vi "eodrecorder_modified.vi"() -> ()   [LabVIEW 2012]
uses:
  eodrecorderstates.ctl
  <vilib>/Utility/error.llb/DialogType.ctl
  <vilib>/_DAQmxBase/Internals/DAQmxBase Create Channel (AI-Voltage-Basic).vi
  <vilib>/_DAQmxBase/Internals/DAQmxBase Timing (Sample Clock).vi
  <vilib>/_DAQmxBase/Internals/DAQmxBase Read (Analog 2D DBL NChan NSamp).vi
panel:
  in  "Channel":tag="Dev1/ai0"
  out "String 2":string
  out "String":string
  out "Tab Control":enum32{"Live Data", "Edit Data", "View Data"}(tab)
  out "WaveformData":T1
  out "# Pretrigger Samples\nAcquired":i32
  out "Pre-Trigger Error Indicator":bool caption="Error Indicator\n(Indicates if trigger occurs before\npre-trigger samples were acquired)"
  in  "Channel Index":i32
  in  "Samples to Read":i32=1000 caption="Samples to Read per Iterartion"
  in  "Pretrigger Samples":i32
  in  "Threshold":dbl
  out "Waveform Graph":dbl[][](graph) caption="Measurement"
  in  "SampleRate":dbl=10000.0
  in  "LiveDataMode":bool
  in  "NumSamptoGrab":i32
  in  "Capture":bool
  in  "Stop":bool
  in  "Open Data":bool
  # "Off"
  # "On"
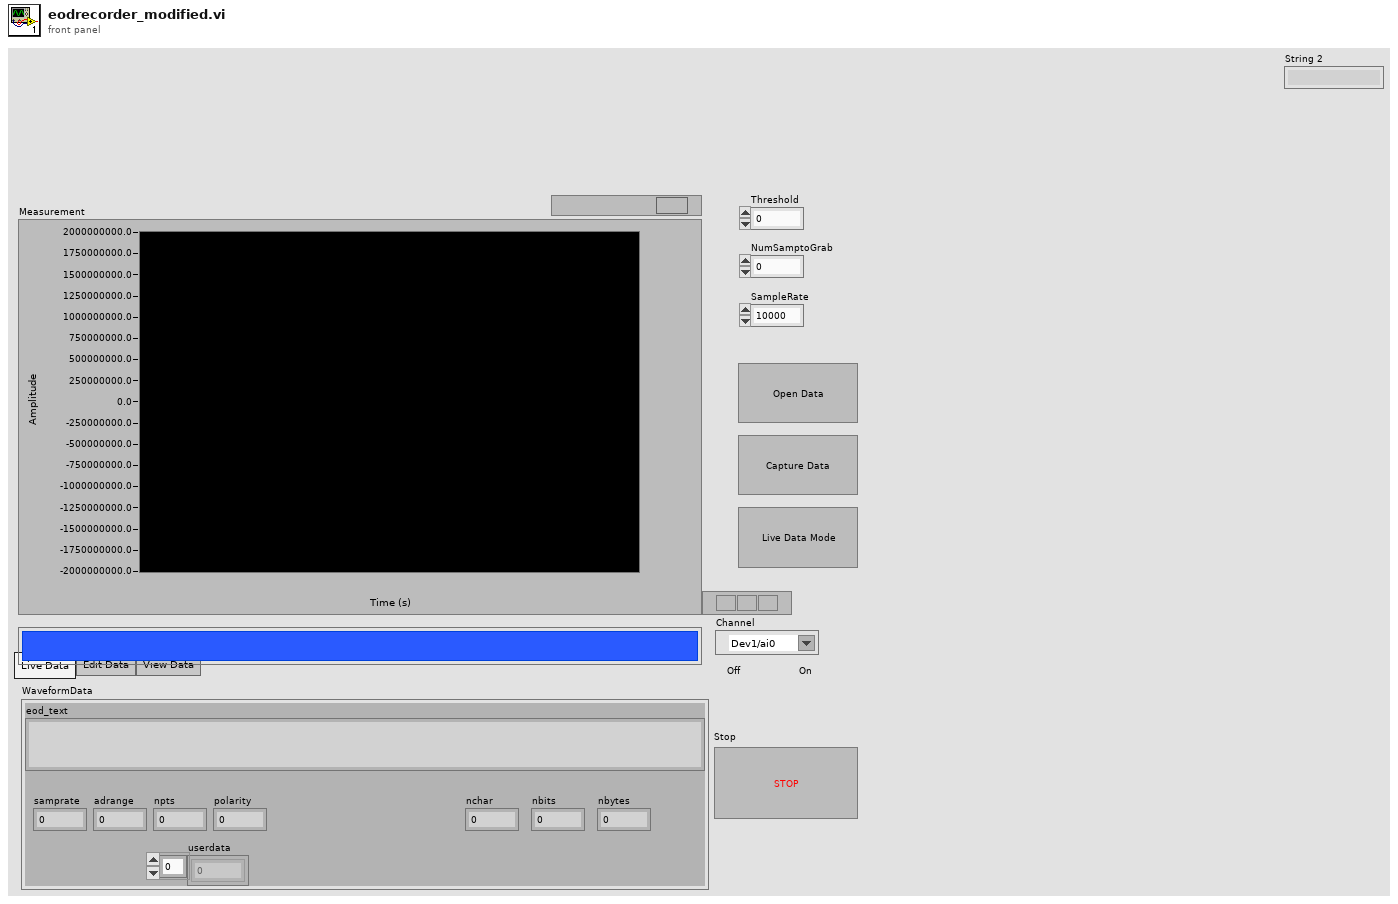
[diagram p1: front panel]
types:
  T1 = cluster{"eod_text":string, "nchar":i32, "nbits":i32, "nbytes":i32, "polarity":i32, "samprate":i32, "adrange":dbl, "userdata":dbl[], "npts":i32, "Wave":dbl[]}
  T2 = cluster{"data":dbl[][], "task ":refnum<k21>, "error ":errorcluster, "Min":dbl, "Max":dbl, "Srate":dbl, "WaveformData":cluster{"eod_text":string, "nchar":i32, "nbits":i32, "nbytes":i32, "polarity":i32, "samprate":i32, "adrange":dbl, "userdata":dbl[], "npts":i32, "Wave":dbl[]}}
  T3 = typedef "eodrecorderstates.ctl" = enum16{"stop", "initialize", "live data", "capture data", "analyze data", "open data", "save data"}
  T4 = enum16{"Rising Edge", "Falling Edge", "Above Level", "Below Level", "When Inside Window", "When Outside Window"}
  T5 = enum16{"open", "replace", "create", "open or create", "replace or create", "replace or create with confirmation"}
  T6 = typedef "DialogType.ctl" = u16
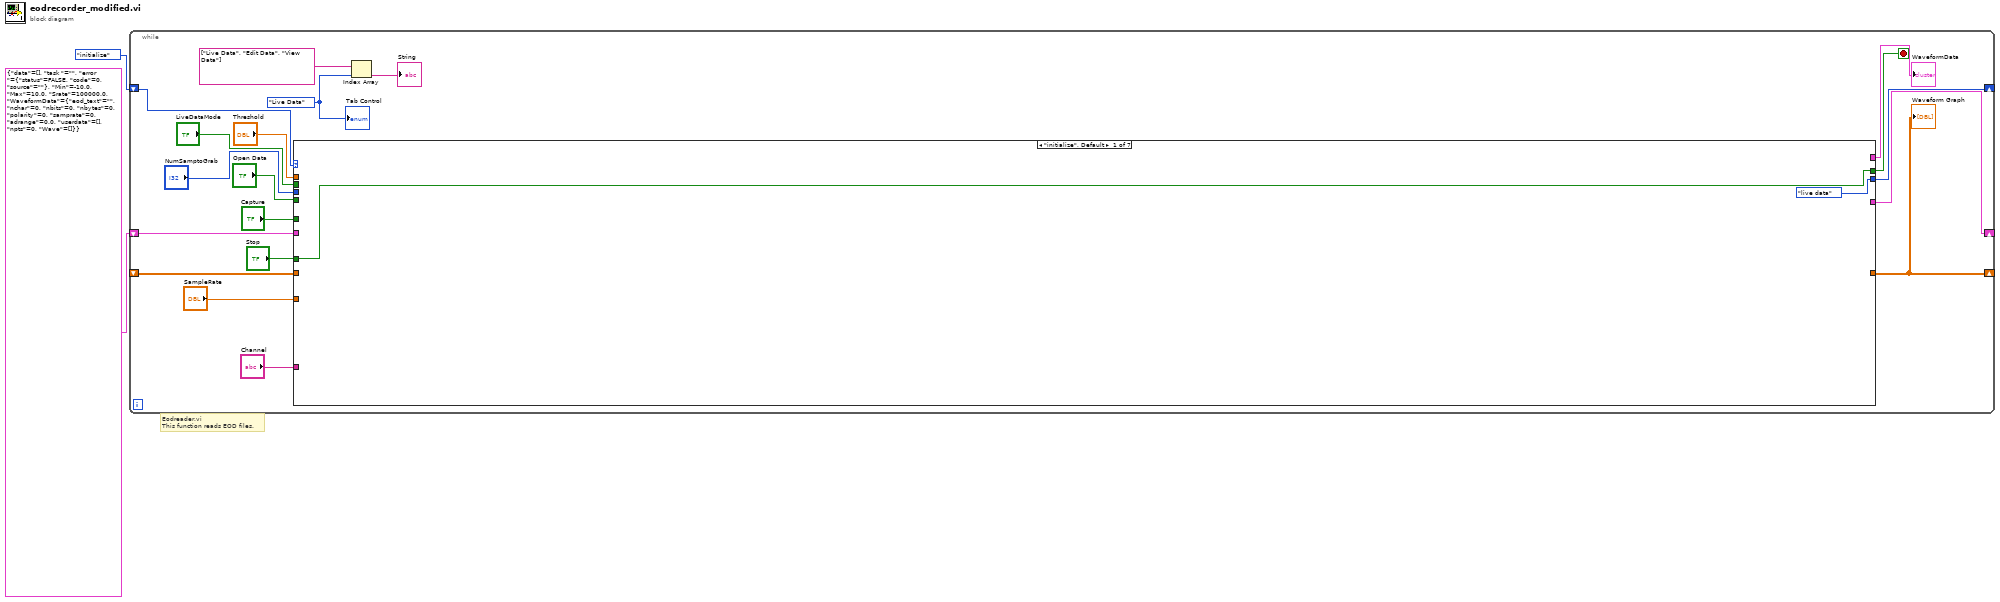
[diagram p0: block diagram]
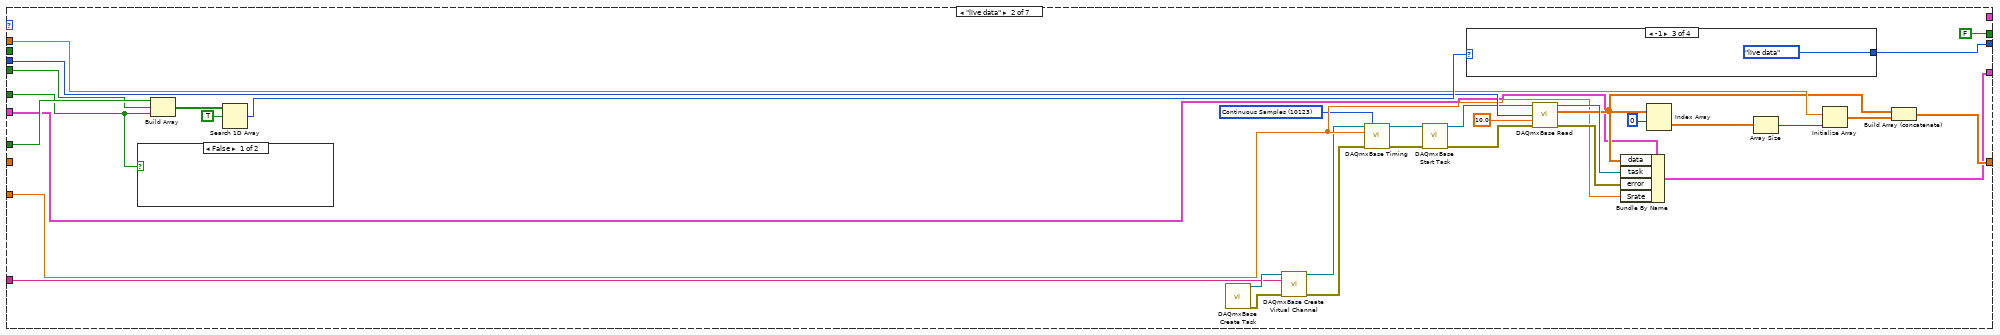
[diagram p2: hidden frame]
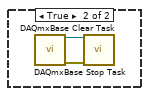
[diagram p3: hidden frame]
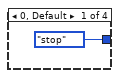
[diagram p4: hidden frame]
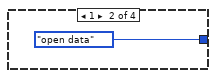
[diagram p5: hidden frame]
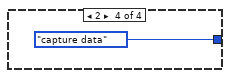
[diagram p6: hidden frame]
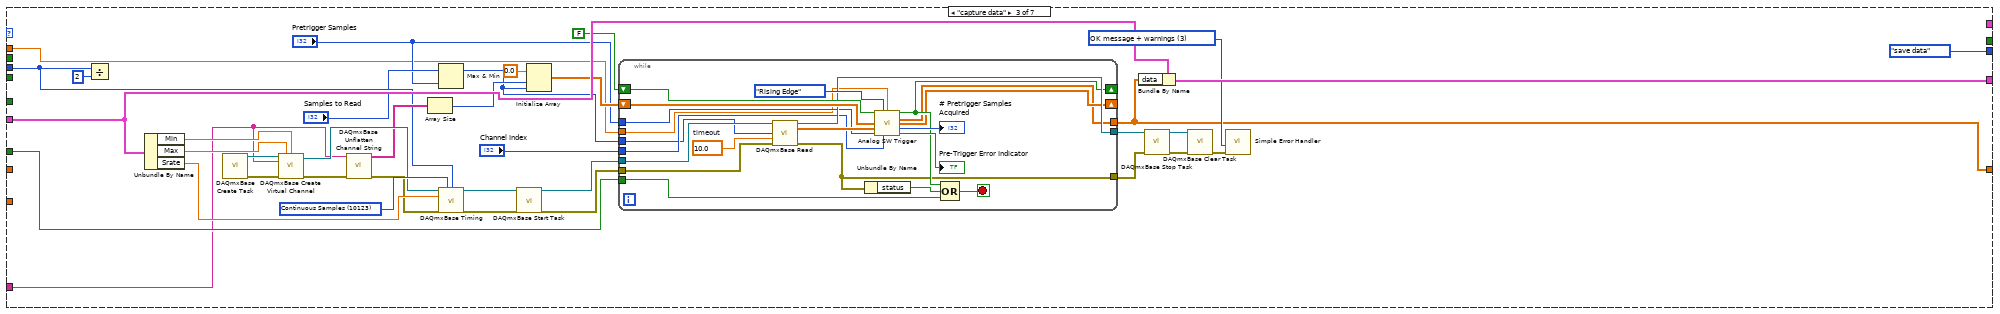
[diagram p7: hidden frame]
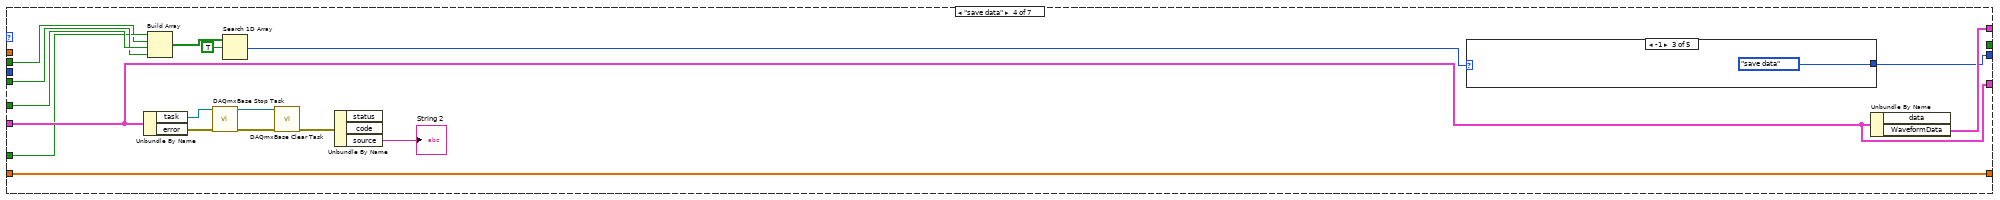
[diagram p8: hidden frame]
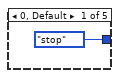
[diagram p9: hidden frame]
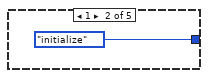
[diagram p10: hidden frame]
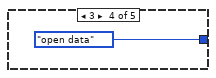
[diagram p11: hidden frame]
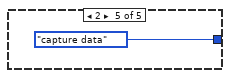
[diagram p12: hidden frame]
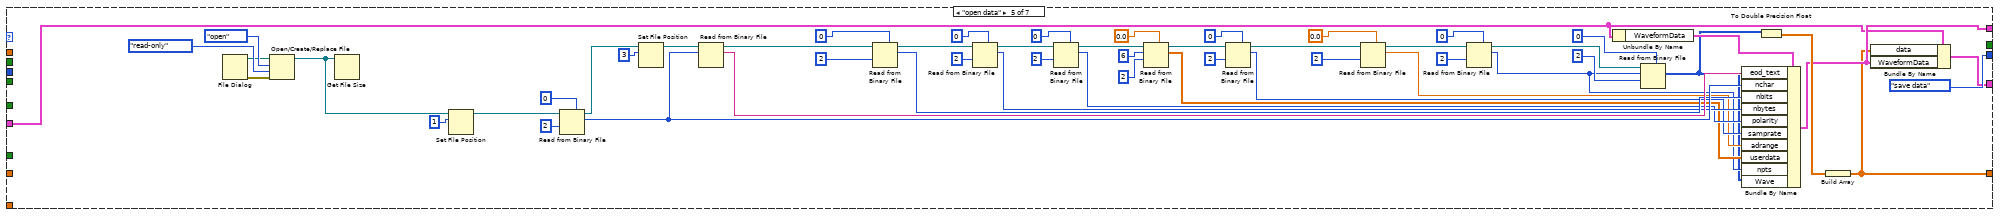
[diagram p13: hidden frame]
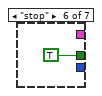
[diagram p14: hidden frame]
diagram:
  # "Eodreader.vi\nThis function reads EOD files."
  n1 = while {
    shift-right: [w20] -> _
    shift-left: eodrecorderstates."initialize" ("Enum") -> [w9]
    shift-right: [w18] -> _
    shift-left: T2 {"data"=[], "task "="", "error "={"status"=FALSE, "code"=0, "source"=""}, "Min"=-10.0, "Max"=10.0, "Srate"=100000.0, "WaveformData"={"eod_text"="", "nchar"=0, "nbits"=0, "nbytes"=0, "polarity"=0, "samprate"=0, "adrange"=0.0, "userdata"=[], "npts"=0, "Wave"=[]}} -> [w15]
    shift-right: [w8] -> _
    shift-left: _ -> [w7]
    stop <- w21 stop-if-true
    w4 = enum32{"Live Data", "Edit Data", "View Data"}."Live Data" ("Tab Control")
    n2 = case shown="\"initialize\", Default" w9 {
      tunnel: [w22 FALSE _ _ _ TRUE _] -> w21
      tunnel: [eodrecorderstates."live data" ("Enum") w54 eodrecorderstates."save data" ("Enum") w134 eodrecorderstates."save data" ("Enum") _ _] -> w20
      tunnel: "Stop" -> [w22 w53 w65 w128 _ _ _]
      tunnel: w15 -> [_ w26 w96 w135 w143 _ _]
      tunnel: [_ w36 w95 w135 w147 _ _] -> w18
      tunnel: [_ _ _ w136 w144 _ _] -> w17
      tunnel: "NumSamptoGrab" -> [_ w46 w81 _ _ _ _]
      tunnel: "SampleRate" -> [_ w35 _ _ _ _ _]
      tunnel: "Open Data" -> [_ w45 _ w130 _ _ _]
      tunnel: "Capture" -> [_ w42 _ w131 _ _ _]
      tunnel: "LiveDataMode" -> [_ _ _ w127 _ _ _]
      tunnel: [_ w43 w63 w120 w142 _ _] -> w8
      tunnel: "Threshold" -> [_ w44 w64 _ _ _ _]
      tunnel: w7 -> [_ _ _ w120 _ _ _]
      tunnel: "Channel" -> [_ w24 w62 _ _ _ _]
      frame "initialize", Default {
      }
      frame "live data" {
        w25 = 10123 items=["Finite Samples"=10178, "Continuous Samples"=10123, "Hardware Timed Single Point"=12522] ("sample mode")
        n3 = case shown="False" w42 {
          frame False {
          }
          frame True {
            n4 = call <vilib>:"DAQmxBase Stop Task.vi"() -> ("task out"=w57:refnum<k21>, "error out"=w56:errorcluster)  [unwired: 14 in]
            n5 = call <vilib>:"DAQmxBase Clear Task.vi"("task in"=w57, "error in"=w56) -> ()  [unwired: 13 in, 1 out]
          }
        }
        n6 = Build Array(w53, w45, w42) -> (w52:bool[])
        n7 = Search 1D Array(1D array=w52, element=TRUE) -> (index of element=w50:i32)  [unwired: 1 in]
        n8 = call <vilib>:"DAQmxBase Create Task.vi"() -> ("task out"=w28:refnum<k21>, "error out"=w27:errorcluster)  [unwired: 5 in, 9 out]
        n9 = call-poly <vilib>:"DAQmxBase Create Virtual Channel.vi"("task in"=w28, "physical channels"=w24, "error in"=w27) -> ("task out"=w34:refnum<k21>, "error out"=w33:errorcluster)  [unwired: 6 in, 5 out]
        n10 = call-poly <vilib>:"DAQmxBase Timing.vi"("task/channels in"=w34, "sample mode"=w25, "rate"=w35, "error in"=w33) -> ("task out"=w32:refnum<k21>, "error out"=w31:errorcluster)  [unwired: 3 in, 7 out]
        n11 = call <vilib>:"DAQmxBase Start Task.vi"("task/channels in"=w32, "error in"=w31) -> ("task out"=w30:refnum<k21>, "error out"=w29:errorcluster)  [unwired: 12 out]
        n12 = case shown="-1" w50 {
          tunnel: [eodrecorderstates."stop" ("Enum") eodrecorderstates."open data" ("Enum") eodrecorderstates."live data" ("Enum") eodrecorderstates."capture data" ("Enum")] -> w54
          frame 0, Default {
          }
          frame 1 {
          }
          frame -1 {
          }
          frame 2 {
          }
        }
        n13 = call-poly <vilib>:"DAQmxBase Read.vi"("task/channels in"=w30, "number of samples per channel"=w46, "timeout"=10.0, "error in"=w29) -> ("task out"=w49:refnum<k21>, "data"=w37:dbl[][], "error out"=w48:errorcluster)  [unwired: 9 out]
        n14 = Bundle By Name(cluster=w26, "data"=w37, "task"=w49, "error"=w48, "Srate"=w35) -> (w36:T2)
        n15 = Index Array(array=w37, index (row)=0) -> (element=w39:dbl[])  [unwired: 1 in]
        n16 = Array Size(array=w39) -> (size(s)=w40:i32)
        n17 = Initialize Array(w44, w40) -> (w38:dbl[])
        n18 = Build Array (concatenate)(w37, w38) -> (w43:dbl[][])
      }
      frame "capture data" {
        w70 = T6 3 items=["no dialog", "OK message", "continue or stop message", "OK message + warnings", "continue/stop + warnings"] ("type of dialog (OK msg:1)")
        w97 = 10123 items=["Finite Samples"=10178, "Continuous Samples"=10123] ("sample mode")
        n19 = Divide(x=w81, y=2) -> ()  [unwired: 1 out]
        n20 = Unbundle By Name(w96) -> ("Min"=w92:dbl, "Max"=w91:dbl, "Srate"=w90:dbl)
        n21 = call <vilib>:"DAQmxBase Create Task.vi"() -> ("task out"=w94:refnum<k21>, "error out"=w93:errorcluster)  [unwired: 14 in]
        n22 = call-poly <vilib>:"DAQmxBase Create Virtual Channel.vi"("task in"=w94, "maximum value"=w91, "minimum value"=w92, "physical channels"=w62, "error in"=w93) -> ("task out"=w89:refnum<k21>, "error out"=w86:errorcluster)  [unwired: 9 in]
        n23 = call "DAQmxBase Unflatten Channel String.vi"("names in"=w62, "error in"=w86) -> ("names out"=w84:string[], "error out"=w85:errorcluster)  [unwired: 12 in]
        n24 = Array Size(array=w84) -> (size(s)=w83:i32)
        n25 = Max & Min(x="Samples to Read", y="Pretrigger Samples") -> (max(x,y)=w72:i32)  [unwired: 1 out]
        n26 = call-poly <vilib>:"DAQmxBase Timing.vi"("task/channels in"=w89, "sample mode"=w97, "samples per channel"=w81, "rate"=w90, "error in"=w85) -> ("task out"=w88:refnum<k21>, "error out"=w87:errorcluster)  [unwired: 2 in, 7 out]
        n27 = call <vilib>:"DAQmxBase Start Task.vi"("task/channels in"=w88, "error in"=w87) -> ("task out"=w78:refnum<k21>, "error out"=w79:errorcluster)  [unwired: 12 out]
        n28 = Initialize Array(0.0, w83, w72) -> (w77:dbl[][])
        n29 = while {
          tunnel: [w110] -> w67
          shift-right: [w109] -> _
          shift-left: FALSE ("Trigger Out") -> [w118]
          shift-right: [w103] -> _
          shift-left: w77 -> [w112]
          tunnel: w79 -> [w108]
          tunnel: w78 -> [w107]
          tunnel: "Pretrigger Samples" -> [w106]
          tunnel: "Channel Index" -> [w105]
          tunnel: w72 -> [w104]
          tunnel: [w102] -> w63
          tunnel: [w101] -> w66
          tunnel: w65 -> [w100]
          tunnel: w64 -> [w99]
          stop <- w116 stop-if-true
          w119 = 10.0  # timeout
          n30 = call-poly <vilib>:"DAQmxBase Read.vi"("task/channels in"=w107, "number of samples per channel"=w104, "timeout"=w119, "error in"=w108) -> ("task out"=w110:refnum<k21>, "data"=w113:dbl[][], "error out"=w101:errorcluster)  [unwired: 9 in]
          n31 = Unbundle By Name(w101) -> ("status"=w117:bool)
          n32 = call "Analog SW Trigger.vi"("Triggered?"=w118, "Condition"=T4."Rising Edge", "Level"=w99, "Initialized Data Array"=w112, "Input Raw Data"=w113, "Pretrigger Samples"=w106, "Index of Condition Channel"=w105) -> ("Trigger Out"=w109:bool, "Output Data (Scaled)"=w102:dbl[][], "Raw Data Out"=w103:dbl[][], "# Pretrigger Samples"=→"# Pretrigger Samples\nAcquired":i32, "Pre-Trigger Error"=→"Pre-Trigger Error Indicator":bool)  [unwired: 4 in]
          n33 = Compound Arithmetic op=OR(w109, w117, w100) -> (w116:bool)
        }
        n34 = Bundle By Name(cluster=w96, "data"=w63) -> (w95:T2)
        n35 = call <vilib>:"DAQmxBase Stop Task.vi"("task/channels in"=w67, "error in"=w66) -> ("task out"=w69:refnum<k21>, "error out"=w68:errorcluster)  [unwired: 12 in]
        n36 = call <vilib>:"DAQmxBase Clear Task.vi"("task in"=w69, "error in"=w68) -> ("error out"=w71:errorcluster)  [unwired: 13 in]
        n37 = call <vilib>:"Simple Error Handler.vi"("type of dialog (OK msg:1)"=w70, "error in (no error)"=w71) -> ()  [unwired: 3 in, 5 out]
      }
      frame "save data" {
        n38 = Unbundle By Name(w135) -> ("task"=w122:refnum<k21>, "error"=w121:errorcluster)
        n39 = Build Array(w128, w127, w131, w130) -> (w133:bool[])
        n40 = call <vilib>:"DAQmxBase Stop Task.vi"("task/channels in"=w122, "error in"=w121) -> ("task out"=w123:refnum<k21>, "error out"=w124:errorcluster)  [unwired: 12 in]
        n41 = Search 1D Array(1D array=w133, element=TRUE) -> (index of element=w129:i32)  [unwired: 1 in]
        n42 = call <vilib>:"DAQmxBase Clear Task.vi"("task in"=w123, "error in"=w124) -> ("error out"=w125:errorcluster)  [unwired: 13 in]
        n43 = Unbundle By Name(w125) -> ("source"=→"String 2":string)  [unwired: 2 out]
        n44 = case shown="-1" w129 {
          tunnel: [eodrecorderstates."stop" ("Enum") eodrecorderstates."initialize" ("Enum") eodrecorderstates."save data" ("Enum") eodrecorderstates."open data" ("Enum") eodrecorderstates."capture data" ("Enum")] -> w134
          frame 0, Default {
          }
          frame 1 {
          }
          frame -1 {
          }
          frame 3 {
          }
          frame 2 {
          }
        }
        n45 = Unbundle By Name(w135) -> ("WaveformData"=w136:T1)  [unwired: 1 out]
      }
      frame "open data" {
        n46 = File Dialog() -> (0:w191:errorcluster, 3:w192:path)  [unwired: 7 in, 2 out]
        n47 = Open/Create/Replace File(file path (use dialog)=w192, error in=w191, operation (0:open)=T5."open", access (0:read/write)=enum16{"read/write", "read-only", "write-only"}."read-only") -> (refnum out=w190:refnum<file>)  [unwired: 2 in, 2 out]
        n48 = Get File Size(file=w190) -> ()  [unwired: 1 in, 3 out]
        n49 = Set File Position(offset (in bytes) (0)=1, refnum=w190) -> (refnum out=w188:refnum<file>)  [unwired: 2 in, 1 out]
        n50 = Read from Binary File(5:u8 0, 9:2, 11:w188) -> (2:w157:u8, 3:w186:refnum<file>)  [unwired: 3 in, 2 out]
        n51 = Set File Position(offset (in bytes) (0)=3, refnum=w186) -> (refnum out=w184:refnum<file>)  [unwired: 2 in, 1 out]
        n52 = Read from Binary File(10:w157, 11:w184) -> (2:w156:string, 3:w183:refnum<file>)  [unwired: 4 in, 2 out]
        n53 = Read from Binary File(5:i8 0, 9:2, 11:w183) -> (2:w155:i8, 3:w159:refnum<file>)  [unwired: 3 in, 2 out]
        n54 = Read from Binary File(5:i8 0, 9:2, 11:w159) -> (2:w154:i8, 3:w160:refnum<file>)  [unwired: 3 in, 2 out]
        n55 = Read from Binary File(5:i8 0, 9:2, 11:w160) -> (2:w153:i8, 3:w158:refnum<file>)  [unwired: 3 in, 2 out]
        n56 = Read from Binary File(5:sgl 0.0, 9:2, 10:6, 11:w158) -> (2:w152:sgl[], 3:w180:refnum<file>)  [unwired: 2 in, 2 out]
        n57 = Read from Binary File(5:u32 0, 9:2, 11:w180) -> (2:w151:u32, 3:w172:refnum<file>)  [unwired: 3 in, 2 out]
        n58 = Read from Binary File(5:sgl 0.0, 9:2, 11:w172) -> (2:w150:sgl, 3:w166:refnum<file>)  [unwired: 3 in, 2 out]
        n59 = Read from Binary File(5:u32 0, 9:2, 11:w166) -> (2:w149:u32, 3:w167:refnum<file>)  [unwired: 3 in, 2 out]
        n60 = Unbundle By Name(w143) -> ("WaveformData"=w148:T1)
        n61 = Read from Binary File(5:0, 9:2, 10:w149, 11:w167) -> (2:w146:i32[])  [unwired: 2 in, 3 out]
        n62 = Bundle By Name(cluster=w148, "eod_text"=w156, "nchar"=w157, "nbits"=w155, "nbytes"=w154, "polarity"=w153, "samprate"=w151, "adrange"=w150, "userdata"=w152, "npts"=w149, "Wave"=w146) -> (w144:T1)
        n63 = To Double Precision Float(number=w146) -> (double precision float=w145:dbl[])
        n64 = Build Array(w145) -> (w142:dbl[][])
        n65 = Bundle By Name(cluster=w143, "data"=w142, "WaveformData"=w144) -> (w147:T2)
      }
      frame "stop" {
      }
      frame "analyze data" {
      }
    }
    "WaveformData" <- w17
    "Waveform Graph" <- w8
    n66 = Index Array(array=string[] ["Live Data", "Edit Data", "View Data"], index=w4) -> (element=→"String":string)
    "Tab Control" <- w4
  }
